vi "Create Evaluation String.vi"(8 "error in (no error)":errorcluster, 10 "Evaluation String":string, 11 "Integer in":refnum<class "Integer.lvclass">) -> (0 "error out":errorcluster, 3 "Integer out":refnum<class "Integer.lvclass">)   [LabVIEW 2018, in "Integer.lvclass"]
uses:
  Integer.lvclass
  Test.lvclass
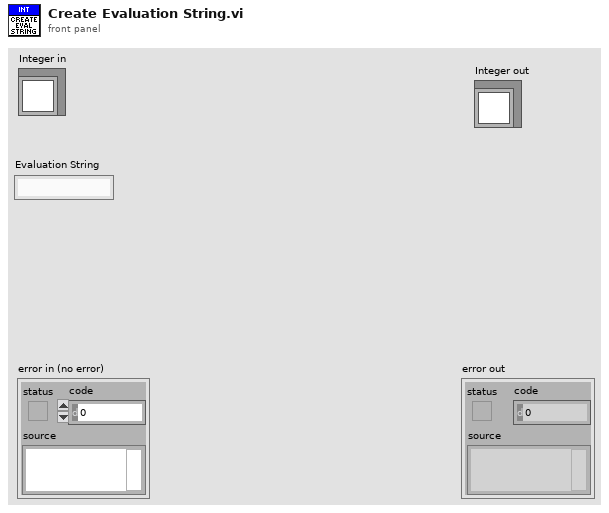
[diagram p1: front panel]
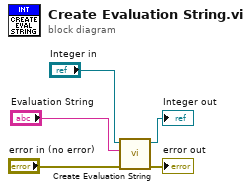
[diagram p0: block diagram]
diagram:
  n1 = call-parent "Create Evaluation String.vi"("error in (no error)"="error in (no error)", "Evaluation String"="Evaluation String", "Test in"="Integer in") -> ("error out"=→"error out":errorcluster, "Test out"=→"Integer out":refnum<class "Integer.lvclass">)  [unwired: 7 in]
